vi "GeraSinalFasor.vi"(0 "params":variant, 2 "Tx Aquisicao":dbl, 4 "estadoIn":variant) -> (15 "sinal":waveform(dbl), 18 "estadoOut":variant)   [LabVIEW 2017]
uses:
  Typedefs/Tipo_ParamsFasor.ctl
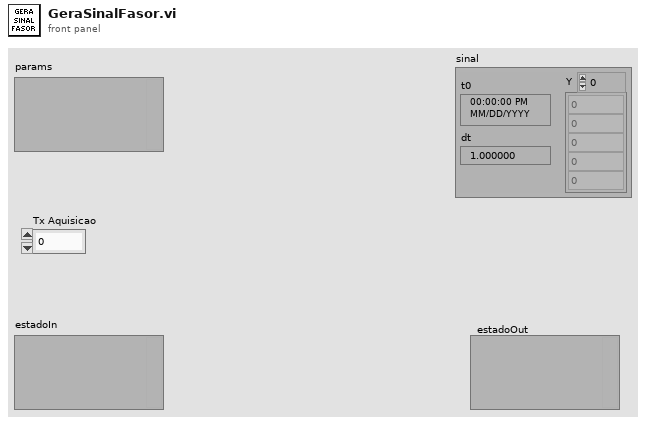
[diagram p1: front panel]
types:
  T1 = typedef "Tipo_ParamsFasor.ctl" = cluster{"Amplitude Repouso":dbl, "Amplitude Pulso":dbl, "Freq. Pulsos":dbl, "Largura Pulsos":dbl}
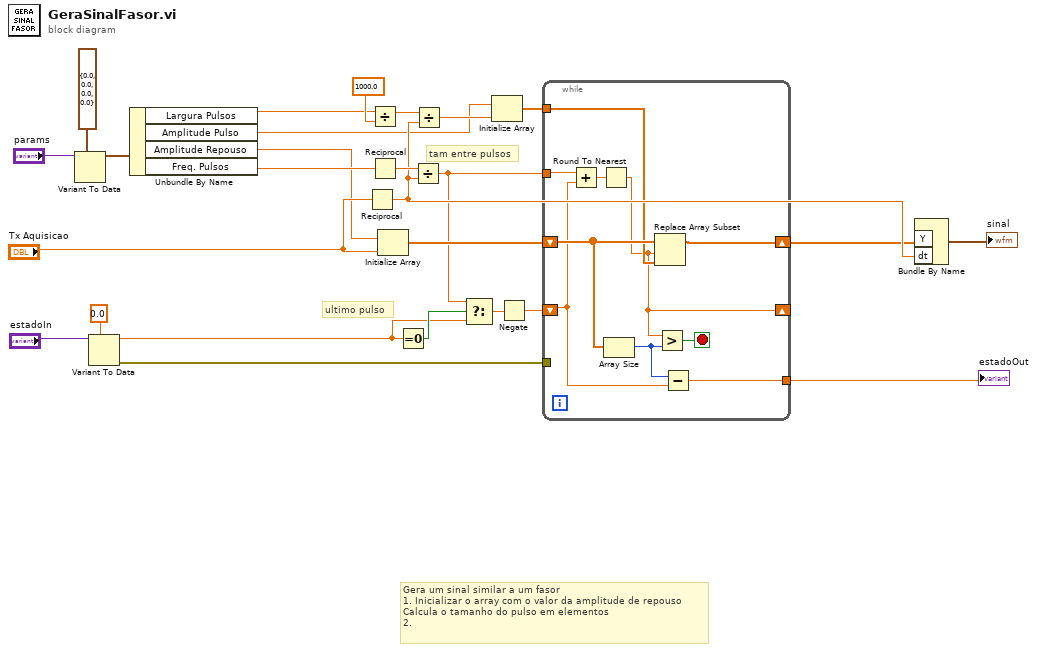
[diagram p0: block diagram]
diagram:
  # "Gera um sinal similar a um fasor\n1. Inicializar o array com o valor da amplitude de repouso \nCalcula o tamanho do pulso em elementos\n2."
  # "ultimo pulso"
  # "tam entre pulsos"
  n1 = Variant To Data(type=T1 {"Amplitude Repouso"=0.0, "Amplitude Pulso"=0.0, "Freq. Pulsos"=0.0, "Largura Pulsos"=0.0} ("Tipo_ParamRuido"), Variant="params") -> (data=w24:T1)  [unwired: 1 in, 1 out]
  n2 = Variant To Data(type=0.0, Variant="estadoIn") -> (data=w3:dbl, error out=w13:errorcluster)  [unwired: 1 in]
  n3 = Unbundle By Name(w24) -> ("Largura Pulsos"=w6:dbl, "Amplitude Pulso"=w7:dbl, "Amplitude Repouso"=w19:dbl, "Freq. Pulsos"=w23:dbl)
  n4 = Reciprocal(x="Tx Aquisicao") -> (1/x=w12:dbl)
  n5 = Divide(x=w6, y=1000.0) -> (x/y=w8:dbl)
  n6 = Reciprocal(x=w23) -> (1/x=w18:dbl)
  n7 = Initialize Array(w19, "Tx Aquisicao") -> (w20:dbl[])
  n8 = Equal To 0?(x=w3) -> (x = 0?=w4:bool)
  n9 = Divide(x=w18, y=w12) -> (x/y=w2:dbl)
  n10 = Divide(x=w8, y=w12) -> (x/y=w11:dbl)
  n11 = Select(t=w2, s=w4, f=w3) -> (s? t:f=w1:dbl)
  n12 = Initialize Array(w7, w11) -> (w10:dbl[])
  n13 = Negate(x=w1) -> (-x=w14:dbl)
  n14 = while {
    tunnel: w2 -> [w36]
    shift-right: [w27] -> _
    shift-left: w14 -> [w31]
    shift-right: [w35] -> w5
    shift-left: w20 -> [w34]
    tunnel: [w30] -> w17
    tunnel: w13 -> [_]
    tunnel: w10 -> [w29]
    stop <- w33 stop-if-true
    n15 = Add(x=w36, y=w31) -> (x+y=w28:dbl)
    n16 = Round To Nearest(number=w28) -> (nearest integer value=w27:dbl)
    n17 = Array Size(array=w34) -> (size(s)=w32:i32)
    n18 = Replace Array Subset(array=w34, new element=w29, index=w27) -> (w35:dbl[])
    n19 = Greater?(x=w27, y=w32) -> (0:w33:bool)
    n20 = Subtract(x=w32, y=w31) -> (x-y=w30:dbl)
  }
  "estadoOut" <- w17
  n21 = Bundle By Name("Y"=w5, "dt"=w12) -> (→"sinal":waveform(dbl))  [unwired: 1 in]
